vi "Queue-base.vi"() -> ()   [LabVIEW 2020]
doc: "Use this template to build a master/slave design pattern. The master loop always executes. It notifies one or more slave loops to execute their code. The slave loop(s) continue executing until they complete, then wait for another notification. Contrast this with the Producer/Consumer pattern in which the consumer loops execute only when they have data in their queue."
panel:
  in  "stop":bool
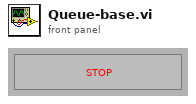
[diagram p1: front panel]
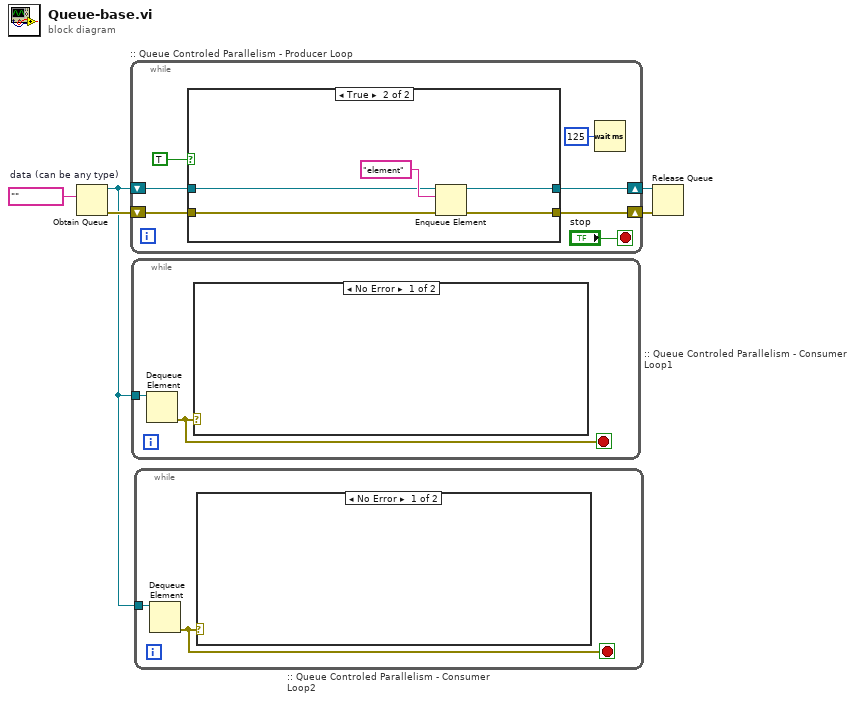
[diagram p0: block diagram]
diagram:
  w1 = ""  # data (can be any type)
  n1 = Obtain Queue(element data type=w1) -> (queue out=w2:refnum<queue>, error out=w5:errorcluster)  [unwired: 4 in, 1 out]
  n2 = while ":: Queue Controled Parallelism - Producer Loop" {
    shift-right: [w10] -> w3
    shift-left: w5 -> [w9]
    shift-right: [w8] -> w4
    shift-left: w2 -> [w11]
    stop <- "stop" stop-if-true
    n3 = case shown="True" TRUE ("Start") {
      tunnel: w11 -> [w14 w16]
      tunnel: [w13 w18] -> w10
      tunnel: w9 -> [w13 w19]
      tunnel: [w14 w15] -> w8
      frame False {
      }
      frame True {
        n4 = Enqueue Element(queue=w16, element="element" ("notification"), error in (no error)=w19) -> (queue out=w15:refnum<queue>, error out=w18:errorcluster)  [unwired: 1 in, 1 out]
      }
    }
    n5 = Wait (ms)(milliseconds to wait=u32 125) -> ()  [unwired: 1 out]
  }
  n6 = while ":: Queue Controled Parallelism - Consumer Loop1" {
    tunnel: w2 -> [w21]
    stop <- w20 stop-if-true
    n7 = Dequeue Element(queue=w21) -> (error out=w20:errorcluster)  [unwired: 2 in, 3 out]
    n8 = case shown="No Error" w20 {
      frame No Error {
      }
      frame Error {
      }
    }
  }
  n9 = while ":: Queue Controled Parallelism - Consumer Loop2" {
    tunnel: w2 -> [w23]
    stop <- w22 stop-if-true
    n10 = Dequeue Element(queue=w23) -> (error out=w22:errorcluster)  [unwired: 2 in, 3 out]
    n11 = case shown="No Error" w22 {
      frame No Error {
      }
      frame Error {
      }
    }
  }
  n12 = Release Queue(queue=w4, error in (no error)=w3) -> ()  [unwired: 1 in, 3 out]
